vi "Servo.vi"(7 "Action":T1, 8 "error in (no error)":errorcluster, 10 "Angle (deg)":i32, 11 "ServoDeviceRef":T2={"DeviceStatus"={"status"=FALSE, "code"=0, "source"=""}, "Digital Module"=enum."Digital Module 1", "PWM Channel"=enum."Invalid", "DeadBand"={"Name"="", "maxPositivePwm"=0, "minPositivePwm"=0, "centerPwm"=0, "maxNegativePwm"=0, "minNegativePwm"=0, "angularRange"=0}}) -> (0 "error out":errorcluster, 2 "Angle (deg)":i32)   [LabVIEW 2013]
uses:
  <vilib>/Rock Robotics/WPI/PWM/Servo/WPI_ServoDeviceRef.ctl
  <vilib>/Rock Robotics/SystemInterfaces/Typedef/FPGA_TypedefDigitalModule.ctl
  <vilib>/Rock Robotics/SystemInterfaces/DIO/FPGA_DIOPWMChannel.ctl
  <vilib>/Rock Robotics/WPI/PWM/WPI_PWMDeadband.ctl
  ServoAction.ctl
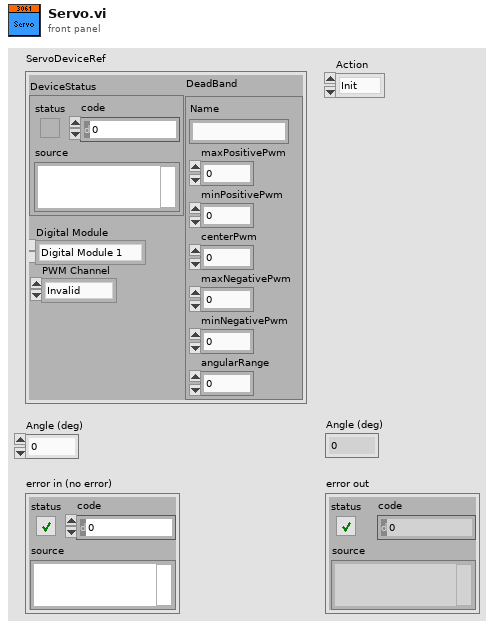
[diagram p1: front panel]
types:
  T1 = typedef "ServoAction.ctl" = enum16{"Init", "SetAngle", "GetAngle", "Disable"}
  T2 = typedef "WPI_ServoDeviceRef.ctl" = cluster{"DeviceStatus":errorcluster, "Digital Module":T3, "PWM Channel":T4, "DeadBand":T5}
  T3 = typedef "FPGA_TypedefDigitalModule.ctl" = enum16{"Digital Module 1", "Digital Module 2"}
  T4 = typedef "FPGA_DIOPWMChannel.ctl" = enum8{"PWM 1", "PWM 2", "PWM 3", "PWM 4", "PWM 5", "PWM 6", "PWM 7", "PWM 8", "PWM 9", "PWM 10", "Invalid"}
  T5 = typedef "WPI_PWMDeadband.ctl" = cluster{"Name":string, "maxPositivePwm":i32, "minPositivePwm":i32, "centerPwm":i32, "maxNegativePwm":i32, "minNegativePwm":i32, "angularRange":u16}
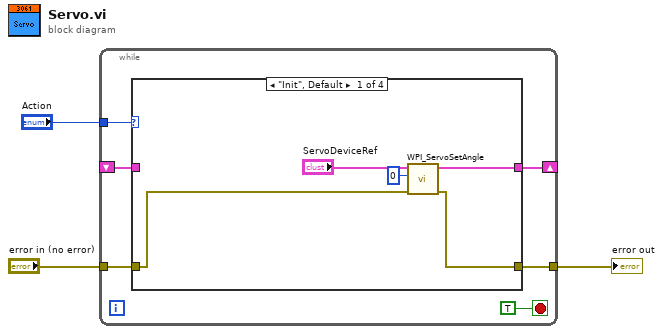
[diagram p0: block diagram]
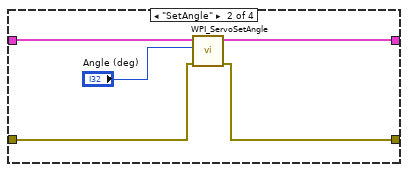
[diagram p2: hidden frame]
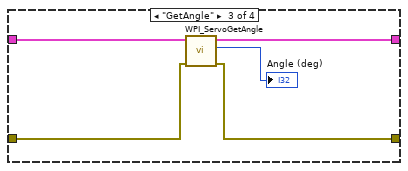
[diagram p3: hidden frame]
diagram:
  n1 = while {
    tunnel: "Action" -> [w8]
    shift-right: [w7] -> _
    shift-left: _ -> [w6]
    tunnel: "error in (no error)" -> [w5]
    tunnel: [w4] -> w1
    stop <- TRUE stop-if-true
    n2 = case shown="\"Init\", Default" w8 {
      tunnel: [w13 w17 w23 w25] -> w7
      tunnel: w6 -> [_ w18 w24 w25]
      tunnel: w5 -> [w11 w16 w22 w26]
      tunnel: [w10 w15 w21 w26] -> w4
      frame "Init", Default {
        n3 = call <vilib>:"WPI_ServoSetAngle.vi"("error in (no error)"=w11, "Angle"=0, "ServoDeviceRef"="ServoDeviceRef") -> ("error out"=w10:errorcluster, "ServoDeviceRef"=w13:T2)  [unwired: 7 in]
      }
      frame "SetAngle" {
        n4 = call <vilib>:"WPI_ServoSetAngle.vi"("error in (no error)"=w16, "Angle"="Angle (deg)", "ServoDeviceRef"=w18) -> ("error out"=w15:errorcluster, "ServoDeviceRef"=w17:T2)  [unwired: 7 in]
      }
      frame "GetAngle" {
        n5 = call <vilib>:"WPI_ServoGetAngle.vi"("ServoDeviceRef"=w24, "error in (no error)"=w22) -> ("ServoDeviceRef"=w23:T2, "Angle"=→"Angle (deg)":u16, "error out"=w21:errorcluster)  [unwired: 6 in]
      }
      frame "Disable" {
      }
    }
  }
  "error out" <- w1
